vi "Get device ID.vi"(8 "error in (no error)":errorcluster, 11 "VISA resource name in":refnum<visa-resource-name>) -> (0 "error out":errorcluster, 2 "ID":string, 3 "VISA Refnum out":refnum<visa-resource-name>)   [LabVIEW 2020, in "Control de MaP.lvlib"]
uses:
  Control de MaP.lvlib
  <vilib>/Instr/_visa.llb/VISA Flush IO Buffer Mask.ctl
  Write--command.vi
panel:
  out "Command out":string
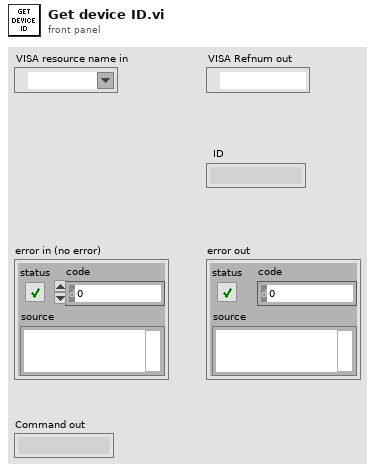
[diagram p1: front panel]
types:
  T1 = typedef "VISA Flush IO Buffer Mask.ctl" = u16
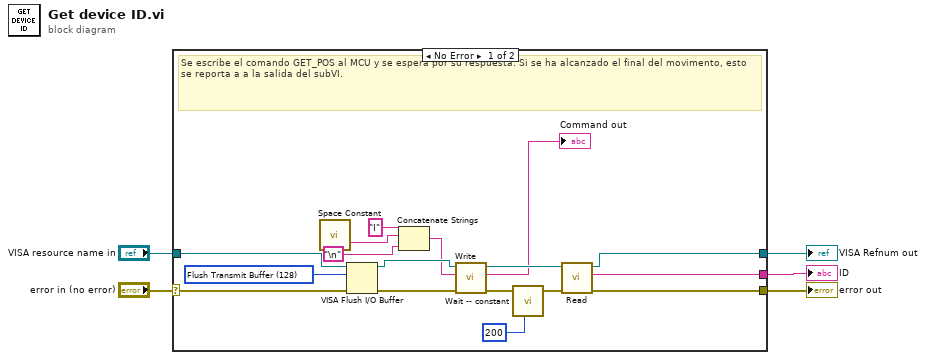
[diagram p0: block diagram]
diagram:
  n1 = case shown="No Error" "error in (no error)" {
    selector: "error in (no error)" -> [w18 w23]
    tunnel: [w7 w23] -> w5
    tunnel: "VISA resource name in" -> [w16 w24]
    tunnel: [w19 w24] -> w2
    tunnel: [w6 _] -> w1
    frame No Error {
      w14 = T1 128 items=["Flush Receive Buffer"=16, "Write Transmit Buffer to Device"=32, "Flush Receive Buffer (No I/O)"=64, "Flush Transmit Buffer"=128] ("Mask")
      # "Se escribe el comando GET_POS al MCU y se espera por su respuesta. Si se ha alcanzado el final del movimento, esto se reporta a a la salida del subVI."
      n2 = call <vilib>:"Space Constant.vi"() -> ("String"=w8:string)
      n3 = VISA Flush I/O Buffer(VISA resource name=w16, mask (16)=w14, error in (no error)=w18) -> (VISA resource name out=w15:refnum<visa-resource-name>, error out=w17:errorcluster)
      n4 = Concatenate Strings("I" ("Command"), w8, "\n") -> (w11:string)
      n5 = call-poly "Write.vi"("error in (no error)"=w17, "Command"=w11, "VISA resource name"=w15) -> ("error out"=w21:errorcluster, "Command out"=→"Command out":string, "VISA resource name out"=w22:refnum<visa-resource-name>)  [unwired: 6 in]
      n6 = call "Wait -- constant.vi"("error in (no error)"=w21, "wait (100 ms)"=u32 200) -> ("error out"=w20:errorcluster)  [unwired: 5 in]
      n7 = call "Read.vi"("error in (no error)"=w20, "VISA resource name"=w22) -> ("error out"=w7:errorcluster, "Recibo de Datos"=w6:string, "VISA resource name out"=w19:refnum<visa-resource-name>)  [unwired: 6 in, 1 out]
    }
    frame Error {
    }
  }
  "error out" <- w5
  "VISA Refnum out" <- w2
  "ID" <- w1
